vi "Keithley 3940 get Ampl.vi"(3 "VISA session":refnum<visa-resource-name>) -> (0 "Stop":bool, 1 "Amplitude":dbl format="%.3e")   [LabVIEW 2020]
doc: "This VI reads the sample and control output of the Lakeshore DRC 93C or 82C temperature controller. The output is an array of the sample and control readings. The input is the numeric GPIB address.\nScott Hannahs, F. Bitter National Magnet Lab, May 1993"
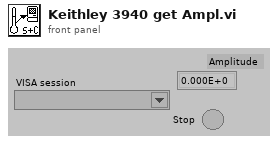
[diagram p1: front panel]
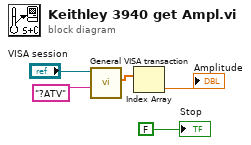
[diagram p0: block diagram]
diagram:
  n1 = call "General VISA transaction.vi"("Command String"="?ATV", "VISA Session"="VISA session") -> ("Measurement"=w5:dbl[])  [unwired: 4 in, 5 out]
  n2 = Index Array(array=w5) -> (element=→"Amplitude":dbl)  [unwired: 1 in]
  "Stop" <- FALSE
